vi "OAT Convert to Even Angle Signal (N Channels).vi"(0 "scaled signals [EU]":waveform(dbl)[](array[waveform]), 1 "analysis method":u16(ring) items=["fast", "accurate"], 2 "reset? (F)":bool, 5 "speed profile":T6 {"speed [RPM]" format="%.2f"; "time [s]" format="%.2f"}, 7 "pulse/revolution (1)":i32=1, 11 "error in (no error)":errorcluster, 12 "max order (auto)":dbl, 13 "zero delay? (F)":bool) -> (4 "even-angle signals":cluster{"r0":dbl, "dr":dbl, "Y":dbl[]}[](array[cluster]) {"r0" format="%.2p"; "dr" format="%.2p"; "Y" format="%.2f"}, 6 "even-angle channel info":T1[](array[typedef]) {"channel info"."pregain" format="%.2f"; "channel info"."weighting filter" items=["Linear", "A-weighting", "B-weighting", "C-weighting", "ITU-R 468-4", "Dolby", "CCITT", "C-message", "Wb", "Wc", "Wd", "We", "Wf", "Wh", "Wj", "Wk", "Wm", "AES17 20 kHz lowpass", "AES17 40 kHz lowpass", "AES17 20 kHz highpass", "AES17 40 kHz highpass"]; "channel info"."dB reference" format="%^.1e"; "channel info"."engineering units" items=["custom..."=0, "V"=1, "A"=21, "C"=30, "pC"=31, "s"=32, "-"=29, "Pa"=2, "N"=20, "g"=3, "m/s^2"=4, "m/s"=5, "m"=6, "mm/s"=12, "mm"=13, "micron/s"=14, "micron"=15, "in/s^2"=7, "in/s"=8, "in"=9, "mil/s"=10, "mil"=11, "rad/s^2"=16, "rad/s"=17, "rad"=18, "deg/s^2"=26, "deg/s"=27, "deg"=28, "RPM"=22, "cycle/s^2"=23, "Hz"=24, "cycle"=25, "strain"=19]; "channel info"."sensor sensitivity" format="%#_5f"}, 8 "even-angle position info":T5, 14 "actual max order":dbl, 15 "error out":errorcluster)   [LabVIEW 2017, in "SoundVib_OrderTracking.lvlib"]
doc: "Converts an even-time-spaced scaled signal to an even-angle-spaced signal by resampling the acquired signal. Wire data to the <B>scaled signal [EU]</B> input to determine the polymorphic instance to use or manually select the instance."
uses:
  <vilib>/addons/Sound and Vibration/Order Analysis/Resample Order Tracking/SoundVib_OrderTracking.lvlib
  <vilib>/addons/Sound and Vibration/Order Analysis/Tach Process/SubVIs/speed profile.ctl
  <vilib>/addons/Sound and Vibration/Order Analysis/Misc/OAT Position Info.ctl
  <vilib>/addons/_NISVFA/_Shared subVIs/Controls/svc_Resampled Channel Info.ctl
  <vilib>/addons/_NISVFA/_Shared subVIs/Controls/svc_Channel Info.ctl
  <vilib>/addons/_NISVFA/_Shared subVIs/Controls/svc_Engineering Units Text Ring.ctl
  <vilib>/addons/_NISVFA/_Shared subVIs/Controls/svc_Weighting Filter Text Ring.ctl
  <vilib>/addons/_NISVFA/_Shared subVIs/Common/svc_Check for Waveform Parameter Continuity (no state).vi
  <vilib>/addons/Sound and Vibration/Order Analysis/Adv Resampling/oa_Adjust Resample State Info.vi
  <vilib>/addons/Sound and Vibration/Order Analysis/Misc/OAT Error Information.vi
  <vilib>/addons/Sound and Vibration/Order Analysis/Adv Resampling/OAT Prepare Resample Data.vi
  <vilib>/addons/_NISVFA/_Shared subVIs/Common/svc_Engineering Units to Unit Label.vi
  <vilib>/addons/_NISVFA/_Shared subVIs/Common/svc_Unit Label to Engineering Units.vi
  <vilib>/addons/Sound and Vibration/Order Analysis/Resample Order Tracking/SoundVib_Resampling.lvlib
  <vilib>/addons/Sound and Vibration/Order Analysis/Tach Process/SoundVib_TachProcess.lvlib
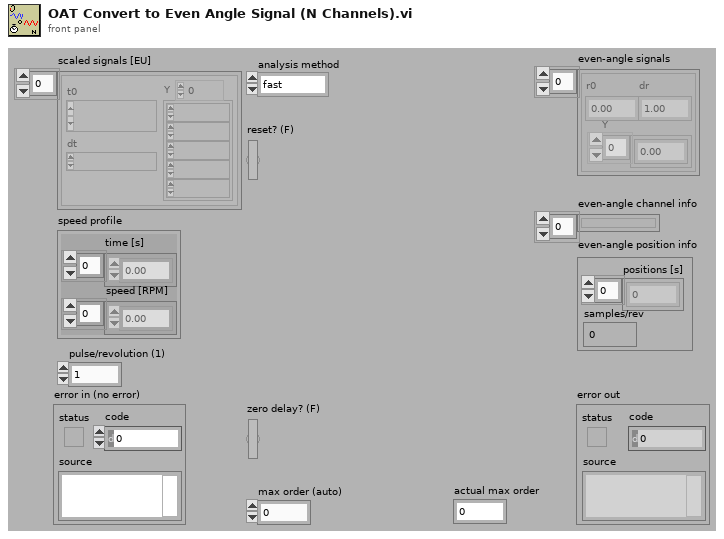
[diagram p1: front panel]
types:
  T1 = typedef "svc_Resampled Channel Info.ctl" = cluster{"channel name":string, "description":string, " channel info":T2}
  T2 = typedef "svc_Channel Info.ctl" = cluster{"sensor sensitivity":dbl, "engineering units":T3, "dB reference":dbl, "custom label":string, "weighting filter":T4, "pregain":dbl}
  T3 = typedef "svc_Engineering Units Text Ring.ctl" = u16
  T4 = typedef "svc_Weighting Filter Text Ring.ctl" = u16
  T5 = typedef "OAT Position Info.ctl" = cluster{"positions [s]":dbl[], "samples/rev":dbl}
  T6 = typedef "SoundVib_TachProcess.lvlib/speed profile.ctl" = cluster{"time [s]":dbl[], "speed [RPM]":dbl[]}
  T7 = cluster{"dt equal":bool, "array length equal":bool, "number channels change":bool}
  T8 = cluster{"dt":bool, "t0 continuity":bool, "array length":bool, "channel info":bool, "name":bool}
  T9 = typedef "OAT Resample Filter Prototype.ctl" = cluster{"left wing":dbl[], "increment":dbl[], "max dec":i32, "timing jitter":enum32{"Interpolation", "Rounding"}, "band limiting?":bool}
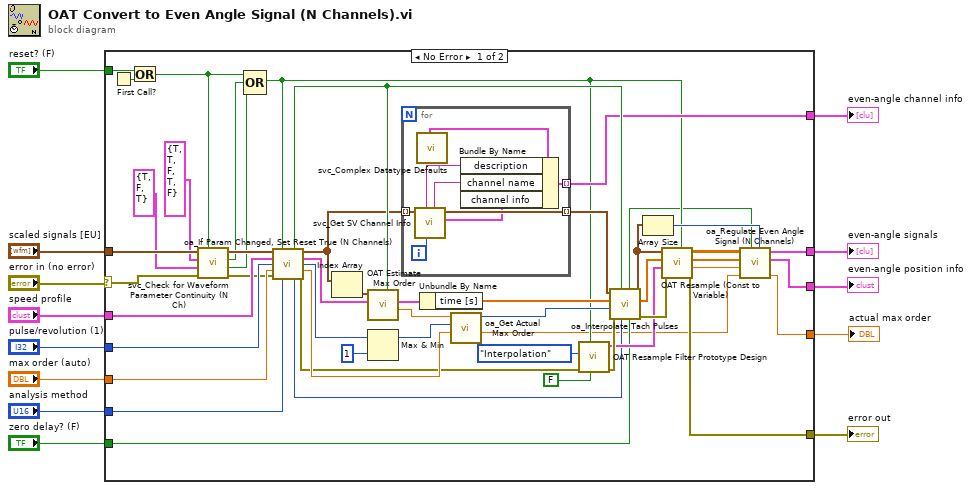
[diagram p0: block diagram]
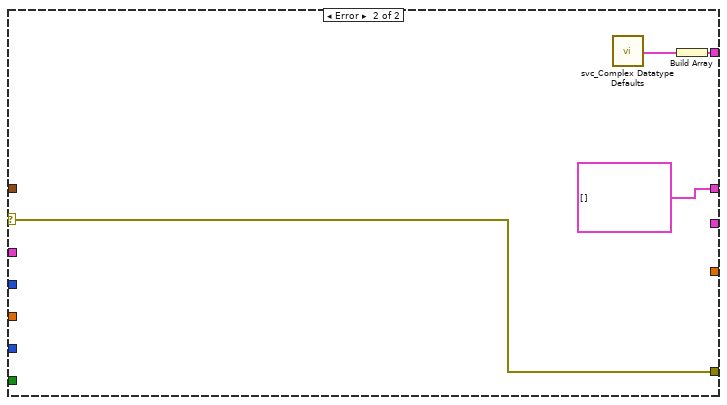
[diagram p2: hidden frame]
diagram:
  n1 = case shown="No Error" "error in (no error)" {
    selector: "error in (no error)" -> [w27 w75]
    tunnel: "pulse/revolution (1)" -> [w49 _]
    tunnel: "max order (auto)" -> [w47 _]
    tunnel: [w19 cluster{dbl, dbl, "Y":dbl[]}[] []] -> w9
    tunnel: "speed profile" -> [w43 _]
    tunnel: [w61 w75] -> w10
    tunnel: "analysis method" -> [w41 _]
    tunnel: [w38 w72] -> w7
    tunnel: [w18 _] -> w6
    tunnel: [w17 _] -> w5
    tunnel: "scaled signals [EU]" -> [w32 _]
    tunnel: "reset? (F)" -> [w44 _]
    tunnel: "zero delay? (F)" -> [w33 _]
    frame No Error {
      n2 = First Call?() -> (First Call?: T/F=w52:bool)
      n3 = Or(x=w44, y=w52) -> (x .or. y?=w30:bool)
      n4 = call <vilib>:"svc_Check for Waveform Parameter Continuity (N Ch).vi"("restart averaging (F)"=w30, "error in (no error)"=w27, "checks for multichannel parameters"=T7 {"dt equal"=TRUE, "array length equal"=FALSE, "number channels change"=TRUE}, "checks for channel parameter change"=T8 {"dt"=TRUE, "t0 continuity"=TRUE, "array length"=FALSE, "channel info"=TRUE, "name"=FALSE}, "scaled signal(s)"=w32) -> ("error out"=w26:errorcluster, "multichannel parameter changed"=w28:bool, "waveform parameter changed"=w29:bool, "dup scaled signal(s)"=w31:waveform(dbl)[])  [unwired: 3 out]
      n5 = Compound Arithmetic op=OR(w30, w29, w28) -> (w24:bool)
      n6 = call <vilib>:"oa_If Param Changed, Set Reset True (N Channels).vi"("scaled signals in [EU]"=w31, "reset in"=w24, "speed profile"=w43, "pulse/revolution in (1)"=w49, "max order in (auto)"=w47, "error in (no error)"=w26, "analysis method in"=w41) -> ("reset out"=w51:bool, "scaled signals out [EU]"=w50:waveform(dbl)[], "speed profile out"=w42:T6, "pulse/revolution out (1)"=w48:i32, "max order out (auto)"=w46:dbl, "analysis method out"=w40:u16, "error out"=w39:errorcluster)  [unwired: 2 in]
      n7 = Index Array(array=w50) -> (element=w56:waveform(dbl))  [unwired: 1 in]
      n8 = call <vilib>:"OAT Estimate Max Order.vi"("reset? (True)"=w51, "speed profile in"=w42, "scaled signal [EU] in"=w56) -> ("max suggested order"=w55:dbl, "speed profile out"=w62:T6)  [unwired: 5 in, 2 out]
      n9 = Max & Min(x=w48, y=1) -> (max(x,y)=w53:i32)  [unwired: 1 out]
      n10 = for {
        tunnel: w50 -> [w71] mode=indexing
        tunnel: [w70] -> w37 mode=indexing
        tunnel: [w68] -> w38 mode=indexing
        i -> [w65]
        n11 = call <vilib>:"svc_Get SV Channel Info.vi"("channel index"=w65, "scaled signal [EU]"=w71) -> ("channel info"=w67:T2, "dup scaled signal [EU]"=w70:waveform(dbl), "channel name"=w64:string, "channel description"=w66:string)  [unwired: 4 in, 2 out]
        n12 = call <vilib>:"svc_Complex Datatype Defaults.vi"() -> ("resampled channel info"=w69:T1)  [unwired: 11 in, 8 out]
        n13 = Bundle By Name(cluster=w69, "description"=w66, "channel name"=w64, "channel info"=w67) -> (w68:T1)
      }
      n14 = Unbundle By Name(w62) -> ("time [s]"=w35:dbl[])
      n15 = call <vilib>:"oa_Get Actual Max Order.vi"("max order (auto)"=w46, "pulse/revolution (1)"=w53, "max suggested order"=w55) -> ("new pulse/revolution"=w20:dbl, "interpolation factor"=w54:i32)  [unwired: 7 in]
      n16 = call <vilib>:"OAT Resample Filter Prototype Design.vi"("alias free"=FALSE ("alias protect in final transition"), "reset? (True)"=w24, "error in (no error)"=w39, "timing jitter"=enum32{"Interpolation", "Rounding"}."Interpolation") -> ("error out"=w60:errorcluster, "filter prototype"=w57:T9)  [unwired: 5 in, 1 out]
      n17 = call <vilib>:"oa_Interpolate Tach Pulses.vi"("zero delay? (F)"=w33, "resolution"=w40, "reset? (True)"=w51, "error in (no error)"=w60, "interpolation factor"=w54, "pulse positions [s]"=w35, "scaled signals (EU)"=w37) -> ("error out"=w59:errorcluster, "interpolated pulse positions[s]"=w34:dbl[], "dup scaled signals (EU)"=w36:waveform(dbl)[], "reset out"=w16:bool)  [unwired: 1 in]
      n18 = Array Size(array=w36) -> (size(s)=w25:i32)
      n19 = call <vilib>:"OAT Resample (Const to Variable).vi"("reset? (True)"=w24, "error in (no error)"=w59, "filter prototype"=w57, "time"=w34, "scaled signals (EU)"=w36) -> ("error out"=w61:errorcluster, "offset"=w21:dbl, "time stamps"=w22:dbl[], "Y"=w23:dbl[][])  [unwired: 3 in]
      n20 = call <vilib>:"oa_Regulate Even Angle Signal (N Channels).vi"("# of ch"=w25, "reset?"=w16, "samples/rev"=w20, "offset"=w21, "time stamps"=w22, "Data"=w23) -> ("actual max order"=w17:dbl, "even-angle position info"=w18:T5, "even-angle signals"=w19:cluster{"r0":dbl, "dr":dbl, "Y":dbl[]}[])  [unwired: 3 in]
    }
    frame Error {
      n21 = call <vilib>:"svc_Complex Datatype Defaults.vi"() -> ("resampled channel info"=w74:T1)  [unwired: 11 in, 8 out]
      n22 = Build Array(w74) -> (w72:T1[])
    }
  }
  "even-angle position info" <- w6
  "error out" <- w10
  "even-angle signals" <- w9
  "even-angle channel info" <- w7
  "actual max order" <- w5
